vi "Find Common Sections.vi"(9 "Offset":u32, 10 "Reference":string, 11 "Target":string) -> (3 "Sections in Reference":T1(array[cluster]))   [LabVIEW 2020]
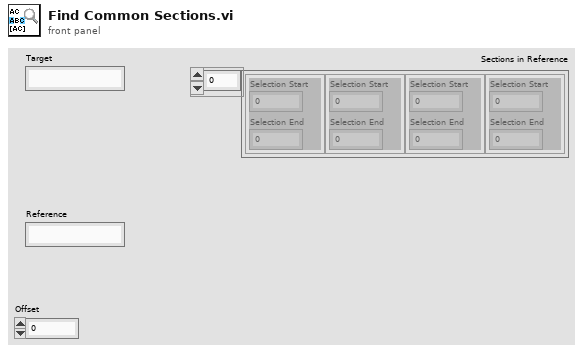
[diagram p1: front panel]
types:
  T1 = cluster{"Selection Start":u32, "Selection End":u32}[]
  T2 = cluster{"Selection Start":u32, "Selection End":u32}
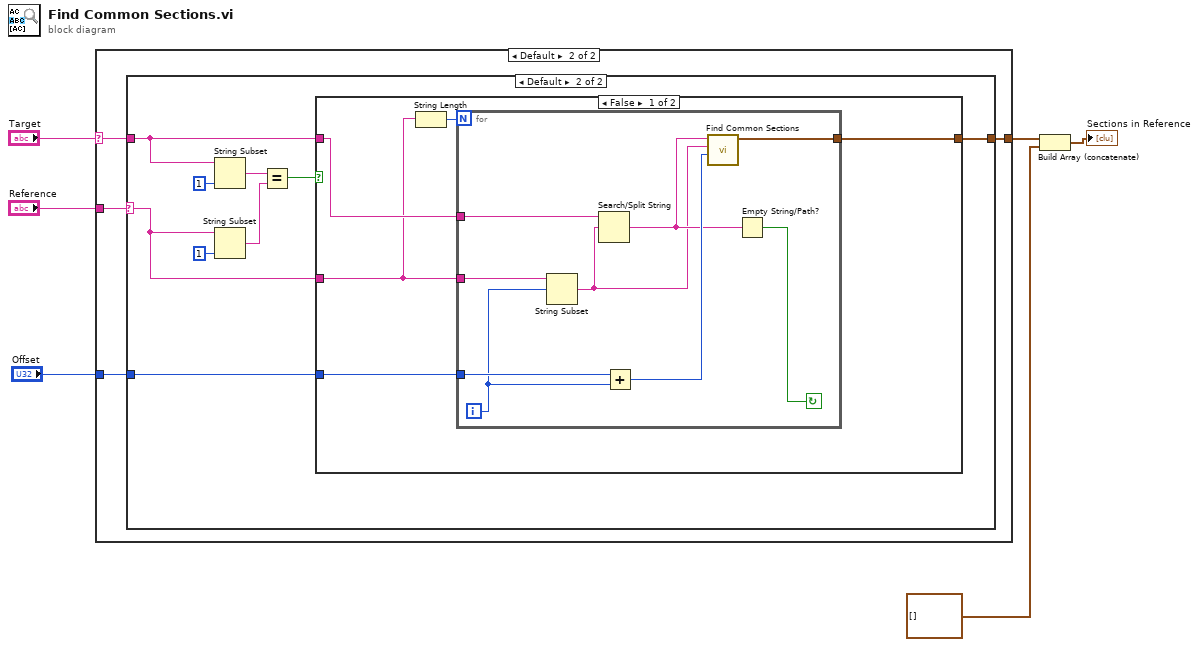
[diagram p0: block diagram]
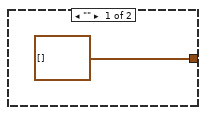
[diagram p2: hidden frame]
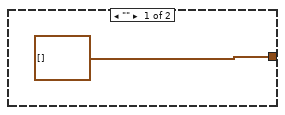
[diagram p3: hidden frame]
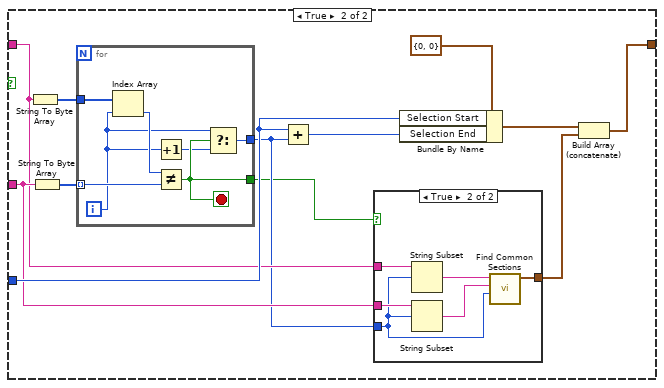
[diagram p4: hidden frame]
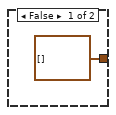
[diagram p5: hidden frame]
diagram:
  n1 = case shown="Default" "Target" {
    selector: "Target" -> [_ w11]
    tunnel: "Reference" -> [_ w10]
    tunnel: "Offset" -> [_ w9]
    tunnel: [T1 [] ("Sections in Reference") w8] -> w6
    frame "" {
    }
    frame Default {
      n2 = case shown="Default" w10 {
        selector: w10 -> [_ w16]
        tunnel: w11 -> [_ w17]
        tunnel: w9 -> [_ w15]
        tunnel: [T1 [] ("Sections in Reference") w13] -> w8
        frame "" {
        }
        frame Default {
          n3 = String Subset(string=w17, length (rest)=1 ("length (rest)")) -> (substring=w19:string)  [unwired: 1 in]
          n4 = String Subset(string=w16, length (rest)=1 ("length (rest)")) -> (substring=w18:string)  [unwired: 1 in]
          n5 = Equal?(x=w19, y=w18) -> (x = y?=w14:bool)
          n6 = case shown="False" w14 {
            tunnel: w17 -> [w25 w39]
            tunnel: w16 -> [w23 w40]
            tunnel: w15 -> [w24 w42]
            tunnel: [w26 w44] -> w13
            frame False {
              n7 = String Length(string=w23) -> (length=w22:i32)
              n8 = for {
                N: w22 -> [_]
                tunnel: [w35] -> w26
                tunnel: w25 -> [w31]
                tunnel: w24 -> [w34]
                tunnel: w23 -> [w33]
                i -> [w29]
                stop <- w32 continue-if-true
                n9 = String Subset(string=w33, offset (0)=w29) -> (substring=w27:string)  [unwired: 1 in]
                n10 = Search/Split String(string=w31, search string/char (-)=w27) -> (match + rest of string=w28:string)  [unwired: 1 in, 2 out]
                n11 = Add(x=w34, y=w29) -> (x+y=w30:u32)
                n12 = call "Find Common Sections.vi"("Offset"=w30, "Reference"=w27, "Target"=w28) -> ("Sections in Reference"=w35:T1)  [unwired: 8 in]
                n13 = Empty String/Path?(string/path=w28) -> (empty?=w32:bool)
              }
            }
            frame True {
              n14 = String To Byte Array(string=w39) -> (unsigned byte array=w46:u8[])
              n15 = String To Byte Array(string=w40) -> (unsigned byte array=w47:u8[])
              n16 = for {
                tunnel: w47 -> [w59] mode=indexing
                tunnel: w46 -> [w61]
                tunnel: [w57] -> w38
                tunnel: [w56] -> w36
                i -> [w58]
                stop <- w56 stop-if-true
                n17 = Index Array(array=w61, index=w58) -> (element=w60:u8)
                n18 = Increment(x=w58) -> (x+1=w55:i32)
                n19 = Not Equal?(x=w60, y=w59) -> (x != y?=w56:bool)
                n20 = Select(t=w58, s=w56, f=w55) -> (s? t:f=w57:i32)
              }
              n21 = Add(x=w42, y=w38) -> (x+y=w37:u32)
              n22 = case shown="True" w36 {
                tunnel: [T1 [] ("Sections in Reference") w54] -> w41
                tunnel: w40 -> [_ w53]
                tunnel: w39 -> [_ w51]
                tunnel: w38 -> [_ w49]
                frame False {
                }
                frame True {
                  n23 = String Subset(string=w51, offset (0)=w49) -> (substring=w50:string)  [unwired: 1 in]
                  n24 = String Subset(string=w53, offset (0)=w49) -> (substring=w52:string)  [unwired: 1 in]
                  n25 = call "Find Common Sections.vi"("Offset"=w49, "Reference"=w52, "Target"=w50) -> ("Sections in Reference"=w54:T1)  [unwired: 8 in]
                }
              }
              n26 = Bundle By Name(cluster=T2 {"Selection Start"=0, "Selection End"=0} ("Sections in Reference"), "Selection Start"=w42, "Selection End"=w37) -> (w43:T2)
              n27 = Build Array (concatenate)(w43, w41) -> (w44:T1)
            }
          }
        }
      }
    }
  }
  n28 = Build Array (concatenate)(w6, T1 [] ("array")) -> (→"Sections in Reference":T1)
